vi "Remove Packet Interference.vi"(11 "Buffer in":u8[](array[numeric])) -> (2 "Filtered?":bool, 3 "Buffer out":u8[](array[numeric]))   [LabVIEW 2015]
doc: "This Vi will be used to filter out cross noise from other transceivers\nIf an A1, A2, A5 or EB command is read that is not an echo (0xFF) or 0x80 then \nthe packet will be removed."
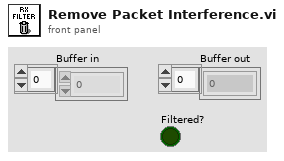
[diagram p1: front panel]
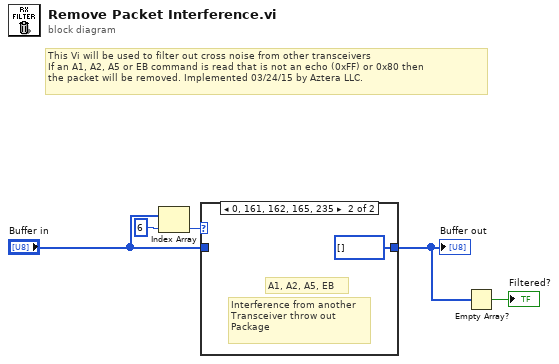
[diagram p0: block diagram]
diagram:
  # "This Vi will be used to filter out cross noise from other transceivers\nIf an A1, A2, A5 or EB command is read that is not an echo (0xFF) or 0x80 then \nthe packet will be removed. Implemented 03/24/15 by Aztera LLC."
  n1 = Index Array(array="Buffer in", index=6) -> (element=w2:u8)
  n2 = case shown="0, 161, 162, 165, 235" w2 {
    tunnel: "Buffer in" -> [w6 _]
    tunnel: [w6 u8[] [] ("Buffer in")] -> w4
    frame Default {
    }
    frame 0, 161, 162, 165, 235 {
      # "Interference from another\nTransceiver throw out \nPackage"
      # "A1, A2, A5, EB"
    }
  }
  "Buffer out" <- w4
  n3 = Empty Array?(array=w4) -> (empty?=→"Filtered?":bool)
